vi "Gradient Dialog.vi"(0 "State In":T2={"Color 1"=0, "Color 2"=0, "Direction"=enum."Top to Bottom", "Frame Color"=16777216, "Fraction"=0.0}, 2 "Control":refnum<vi>) -> (4 "State Out":T2={"Color 1"=0, "Color 2"=0, "Direction"=enum."Top to Bottom", "Frame Color"=16777216, "Fraction"=0.0})   [LabVIEW 2020, in "KBackground Gradient.xctl"]
uses:
  KBackground Gradient.xctl
  State.vi
  Buttons/KCheckmarkBoolean 2.ctl
panel:
  out "exit":bool
  in  "Preview":T1
  in  "Cancel Button":bool
  in  "OK Button":bool
  in  "Frame Color":u32(colorbox)=16777216
  in  "Direction":T3(ring)
  in  "Slide":dbl(slide) scale=0.0..1.0
  in  "Color 2":u32(colorbox)
  in  "Color 1":u32(colorbox)
  out "Color Ramp":i32[][](graph)
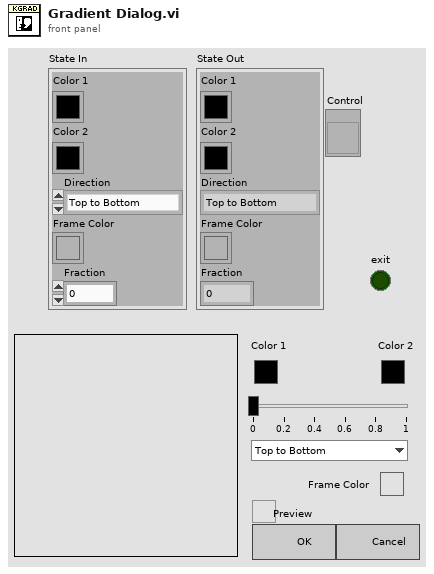
[diagram p1: front panel]
types:
  T1 = typedef "KCheckmarkBoolean 2.ctl" = bool
  T2 = typedef "KBackground Gradient.xctl/State.vi" = cluster{"Color 1":u32, "Color 2":u32, "Direction":enum16{"Top to Bottom", "Bottom to Top", "Left to Right", "Right to Left"}, "Frame Color":u32, "Fraction":dbl}
  T3 = enum16{"Top to Bottom", "Bottom to Top", "Left to Right", "Right to Left"}
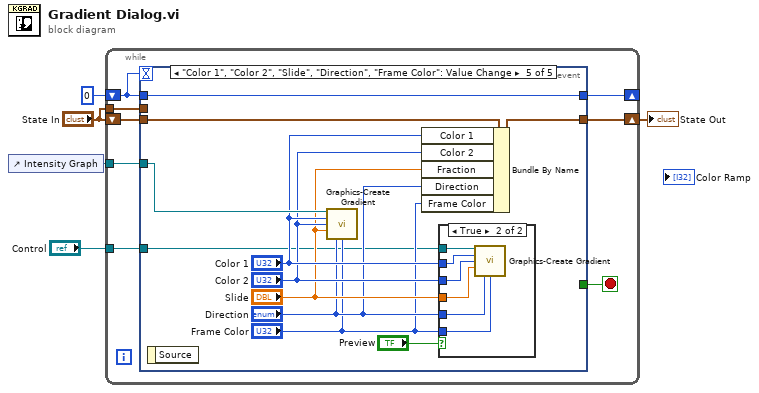
[diagram p0: block diagram]
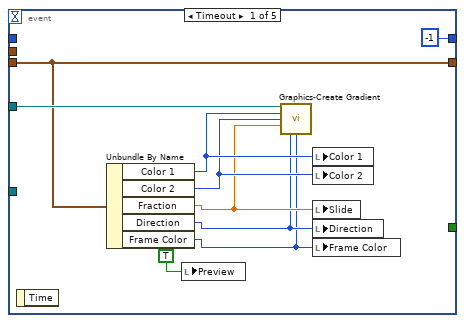
[diagram p2: hidden frame]
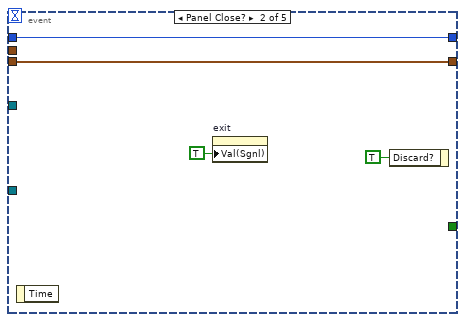
[diagram p3: hidden frame]
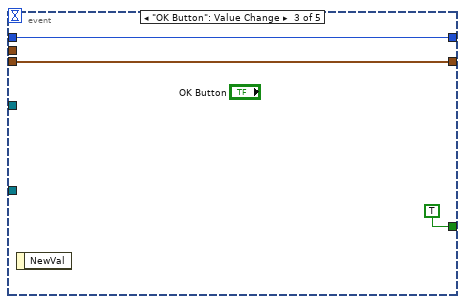
[diagram p4: hidden frame]
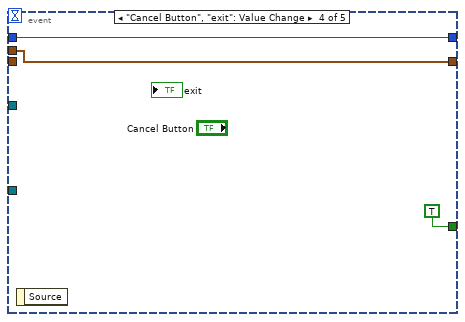
[diagram p5: hidden frame]
diagram:
  n1 = control-ref of="Intensity Graph"() -> (w4:refnum<vi>)
  n2 = while {
    shift-right: [w11] -> _
    shift-left: 0 -> [w12]
    tunnel: w4 -> [w10]
    shift-right: [w8] -> w3
    shift-left: "State In" -> [w9]
    tunnel: "State In" -> [w7]
    tunnel: "Control" -> [w6]
    stop <- w13 stop-if-true
    n3 = event shown="[4] \"Color 1\", \"Color 2\", \"Slide\", \"Direction\", \"Frame Color\": Value Change" {
      selector: _ -> [_ _ _ _ _]
      dyn-events: _ -> [_ _ _ _ _]
      timeout: w12 -> [_ _ _ _ _]
      tunnel: [_ _ TRUE ("stop") TRUE ("stop") _] -> w13
      tunnel: w12 -> [_ w26 w29 w32 w43]
      tunnel: [-1 w26 w29 w32 w43] -> w11
      tunnel: w10 -> [w21 _ _ _ w42]
      tunnel: w9 -> [w20 w25 w28 _ w41]
      tunnel: [w20 w25 w28 w31 w40] -> w8
      tunnel: w7 -> [_ _ _ w31 _]
      tunnel: w6 -> [_ _ _ _ w33]
      event Timeout {
        n4 = event-data() -> ()  [unwired: 1 in, 1 out]
        n5 = Unbundle By Name(w20) -> ("Color 1"=w19:u32, "Color 2"=w18:u32, "Fraction"=w17:dbl, "Direction"=w16:T3, "Frame Color"=w15:u32)
        n6 = local write "Preview"(T1 TRUE ("Preview")) -> ()
        n7 = call "Graphics-Create Gradient.vi"("intensity graph"=w21, "Color 1"=w19, "Color 2"=w18, "Fraction"=w17, "Direction"=w16, "Frame Color"=w15) -> ()  [unwired: 9 in, 1 out]
        n8 = local write "Color 1"(w19) -> ()
        n9 = local write "Color 2"(w18) -> ()
        n10 = local write "Slide"(w17) -> ()
        n11 = local write "Direction"(w16) -> ()
        n12 = local write "Frame Color"(w15) -> ()
      }
      event Panel Close? {
        n13 = event-data() -> ()  [unwired: 1 in, 1 out]
        n14 = property on="exit" class="Bool (strict)"("Val(Sgnl)"=TRUE ("Value (Signaling)")) -> ()  [unwired: 2 in, 2 out]
        n15 = event-data("Discard?"=TRUE) -> ()  [unwired: 1 in, 1 out]
      }
      event "OK Button": Value Change {
        n16 = event-data() -> ()  [unwired: 1 in, 1 out]
      }
      event "Cancel Button", "exit": Value Change {
        n17 = event-data() -> ()  [unwired: 1 in, 1 out]
      }
      event "Color 1", "Color 2", "Slide", "Direction", "Frame Color": Value Change {
        n18 = event-data() -> ()  [unwired: 1 in, 1 out]
        n19 = call "Graphics-Create Gradient.vi"("intensity graph"=w42, "Color 1"="Color 1", "Color 2"="Color 2", "Fraction"="Slide", "Direction"="Direction", "Frame Color"="Frame Color") -> ()  [unwired: 9 in, 1 out]
        n20 = Bundle By Name(cluster=w41, "Color 1"="Color 1", "Color 2"="Color 2", "Fraction"="Slide", "Direction"="Direction", "Frame Color"="Frame Color") -> (w40:T2)
        n21 = case shown="True" "Preview" {
          tunnel: "Color 1" -> [_ w48]
          tunnel: "Color 2" -> [_ w47]
          tunnel: "Slide" -> [_ w46]
          tunnel: "Direction" -> [_ w45]
          tunnel: "Frame Color" -> [_ w44]
          tunnel: w33 -> [_ w49]
          frame False {
          }
          frame True {
            n22 = call "Graphics-Create Gradient.vi"("intensity graph"=w49, "Color 1"=w48, "Color 2"=w47, "Fraction"=w46, "Direction"=w45, "Frame Color"=w44) -> ()  [unwired: 9 in, 1 out]
          }
        }
      }
    }
  }
  "State Out" <- w3
